vi "host.vi"() -> ()   [LabVIEW 2020]
uses:
  <vilib>/DAQmx/write.llb/DAQmx Write (Analog Wfm 1Chan NSamp).vi
  <vilib>/DAQmx/create/channels.llb/DAQmx Create Channel (AO-Voltage-Basic).vi
  <vilib>/DAQmx/configure/timing.llb/DAQmx Timing (Sample Clock).vi
  <vilib>/DAQmx/miscellaneous.llb/DAQmx Fill In Error Info.vi
  <vilib>/Utility/file.llb/Write Delimited Spreadsheet (DBL).vi
  <resource>/objmgr/daqmx.rc
panel:
  out "time":dbl
  in  "y predict save":path
  out "max iteration":dbl
  out "X":dbl[][](array[numeric])
  in  "X data filepath":path
  out "y waveform":cluster{"Numeric":dbl, "Double":dbl}(graph)
  in  "stop":bool
  out "iteration":dbl
  out "y predict values":dbl[](array[numeric])
  out "y":dbl[][](array[numeric])
  in  "y data filepath":path
  out "Waveform Graph":dbl[][](graph)
  out "t":dbl[][](array[numeric])
  in  "t data filepath":path
  out "size":dbl
  in  "error in":errorcluster
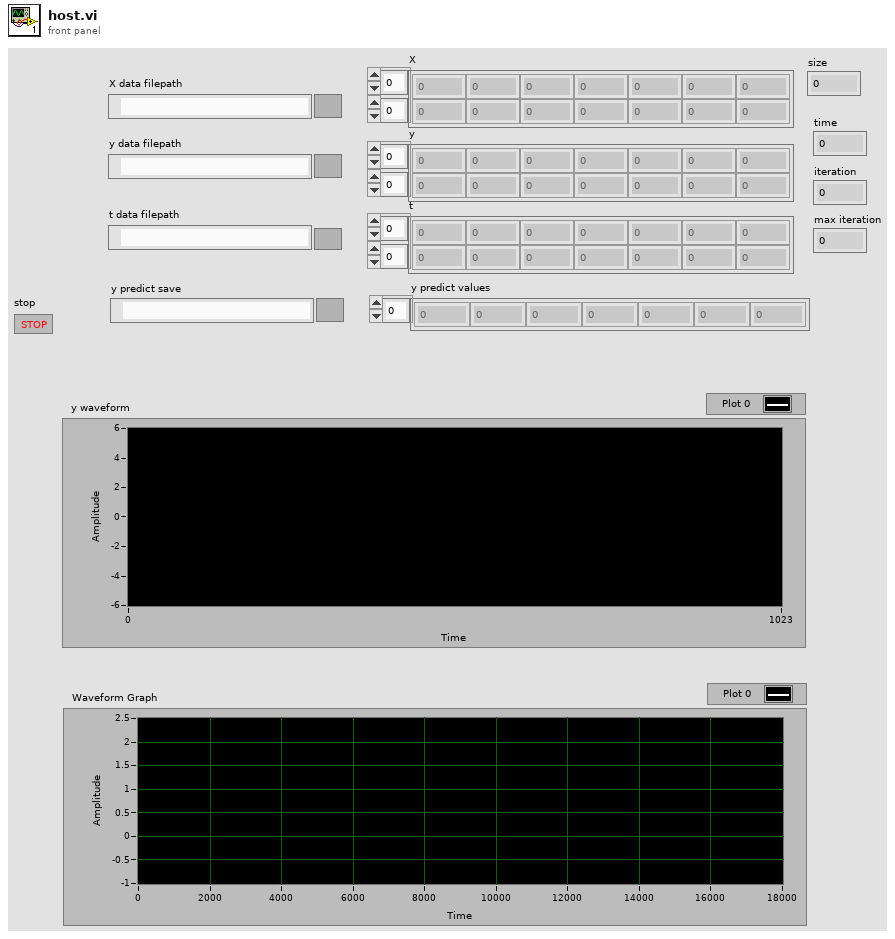
[diagram p1: front panel]
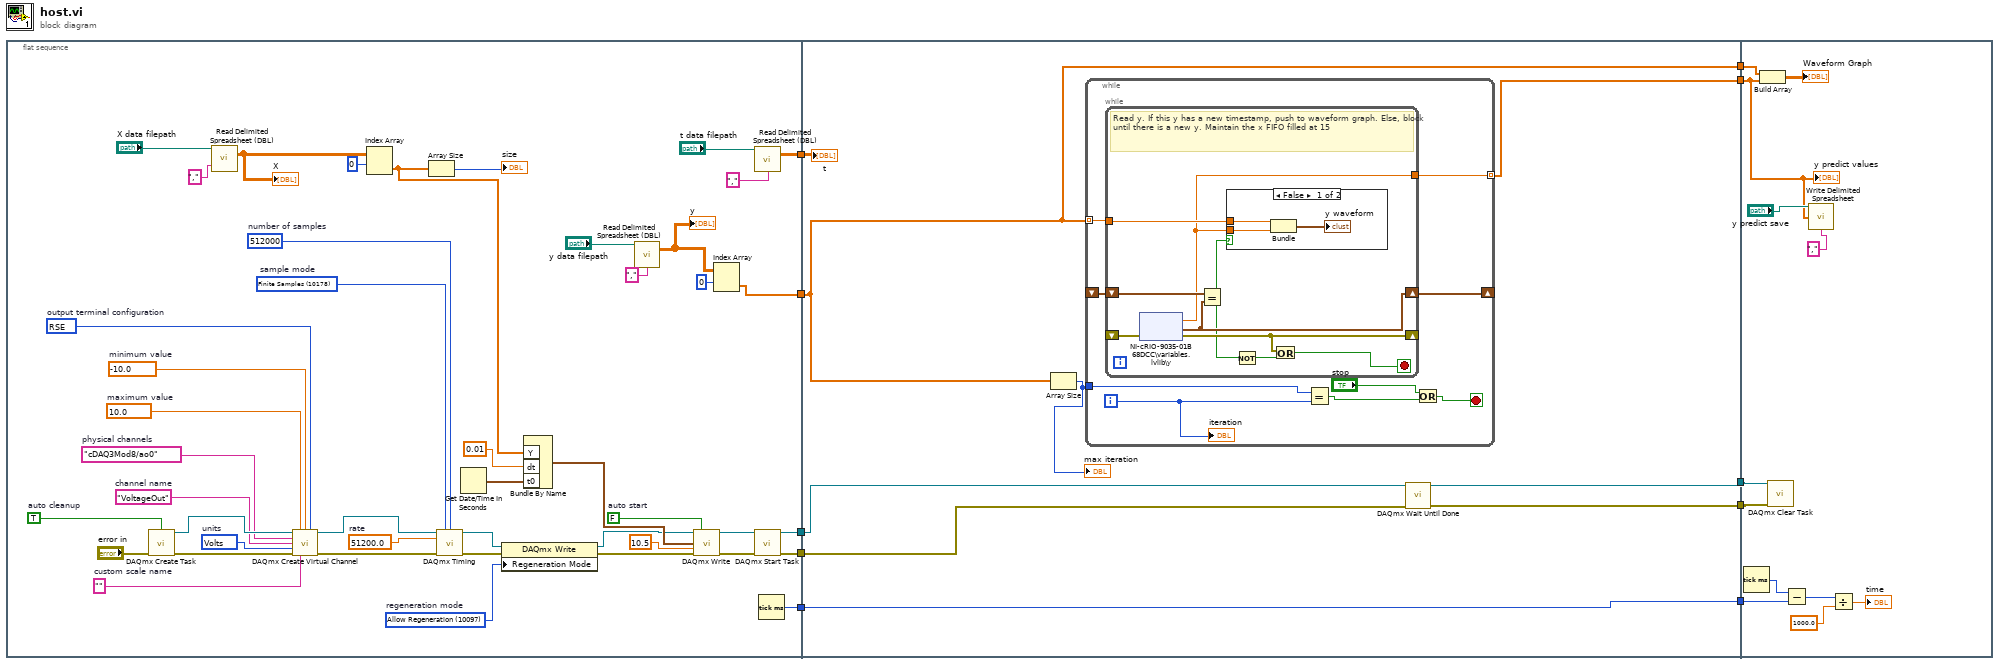
[diagram p0: block diagram]
diagram:
  n1 = flat-sequence {
    tunnel: [w53] -> w10
    tunnel: [w14] -> w9
    tunnel: [w13] -> w8
    tunnel: [w12] -> w6
    tunnel: [w11] -> w5
    tunnel: w10 -> [w64]
    tunnel: w9 -> [w56]
    tunnel: w8 -> [w57]
    tunnel: [w59] -> w7
    tunnel: w6 -> [w60]
    tunnel: w5 -> [w62]
    tunnel: [w62] -> w4
    tunnel: [w61] -> w3
    tunnel: [w60] -> w2
    tunnel: [w58] -> w1
    tunnel: w7 -> [w97]
    tunnel: w4 -> [w94]
    tunnel: w3 -> [w87]
    tunnel: w2 -> [w90]
    tunnel: w1 -> [w96]
    frame #0 {
      w21 = tag "cDAQ3Mod8/ao0"  # physical channels
      w26 = 512000  # number of samples
      w28 = 10097 items=["Allow Regeneration"=10097, "Do Not Allow Regeneration"=10158]  # regeneration mode
      w27 = 10178 items=["Finite Samples"=10178, "Continuous Samples"=10123, "Hardware Timed Single Point"=12522]  # sample mode
      w25 = 51200.0  # rate
      w22 = 10083 items=["Default"=-1, "RSE"=10083, "Differential"=10106, "Pseudodifferential"=12529]  # output terminal configuration
      w19 = 10348 items=["Volts"=10348, "From Custom Scale"=10065]  # units
      w20 = "VoltageOut"  # channel name
      w18 = ""  # custom scale name
      w23 = -10.0  # minimum value
      w24 = 10.0  # maximum value
      w17 = TRUE  # auto cleanup
      w16 = FALSE  # auto start
      n2 = call <vilib>:"DAQmx Create Task.vi"("auto cleanup"=w17, "error in"="error in") -> ("task out"=w34:refnum<k21>, "error out"=w33:errorcluster)  [unwired: 12 in]
      n3 = call <vilib>:"Read Delimited Spreadsheet (DBL).vi"("file path (dialog if empty)"="X data filepath", "delimiter (\\t)"=",") -> ("all rows"=w47:dbl[][])  [unwired: 8 in, 5 out]
      "X" <- w47
      n4 = call-poly <vilib>:"DAQmx Create Virtual Channel.vi"("task in"=w34, "maximum value"=w24, "minimum value"=w23, "output terminal configuration"=w22, "physical channels"=w21, "name to assign"=w20, "units"=w19, "error in"=w33, "custom scale name"=w18) -> ("task out"=w37:refnum<k21>, "error out"=w35:errorcluster)  [unwired: 5 in]
      n5 = Index Array(array=w47, index (row)=0) -> (element=w48:dbl[])  [unwired: 1 in]
      n6 = Array Size(array=w48) -> (size(s)=→"size":i32)
      n7 = call-poly <vilib>:"DAQmx Timing.vi"("task/channels in"=w37, "sample mode"=w27, "samples per channel"=w26, "rate"=w25, "error in"=w35) -> ("task out"=w38:refnum<k21>, "error out"=w36:errorcluster)  [unwired: 9 in]
      n8 = Get Date/Time In Seconds() -> (seconds since 1Jan1904=w43:timestamp)
      n9 = property class="DAQmx Write"(reference=w38, error in=w36, "Regeneration Mode"=w28) -> (reference out=w39:refnum<k21>, error out=w40:errorcluster)
      n10 = Bundle By Name("Y"=w48, "dt"=0.01, "t0"=w43) -> (w44:waveform(dbl))  [unwired: 1 in]
      n11 = call <vilib>:"Read Delimited Spreadsheet (DBL).vi"("file path (dialog if empty)"="y data filepath", "delimiter (\\t)"=",") -> ("all rows"=w51:dbl[][])  [unwired: 8 in, 5 out]
      "y" <- w51
      n12 = call-poly <vilib>:"DAQmx Write.vi"("task/channels in"=w39, "auto start"=w16, "data"=w44, "timeout"=10.5, "error in"=w40) -> ("task out"=w41:refnum<k21>, "error out"=w42:errorcluster)  [unwired: 8 in, 1 out]
      n13 = Index Array(array=w51, index (row)=0) -> (element=w12:dbl[])  [unwired: 1 in]
      n14 = call <vilib>:"Read Delimited Spreadsheet (DBL).vi"("file path (dialog if empty)"="t data filepath", "delimiter (\\t)"=",") -> ("all rows"=w53:dbl[][])  [unwired: 8 in, 5 out]
      n15 = call <vilib>:"DAQmx Start Task.vi"("task/channels in"=w41, "error in"=w42) -> ("task out"=w14:refnum<k21>, "error out"=w13:errorcluster)  [unwired: 12 in]
      n16 = Tick Count (ms)() -> (millisecond timer value=w11:u32)
    }
    frame #1 {
      n17 = Array Size(array=w60) -> (size(s)=w63:i32)
      "max iteration" <- w63
      n18 = while {
        tunnel: w60 -> [w73] mode=indexing
        tunnel: [w70] -> w61 mode=indexing
        shift-right: [w72] -> _
        shift-left: _ -> [w71]
        tunnel: w63 -> [w69]
        i -> [w65]
        stop <- w67 stop-if-true
        n19 = while {
          shift-right: [w81] -> w72
          shift-left: w71 -> [w80]
          shift-right: [w79] -> _
          shift-left: _ -> [w82]
          tunnel: w73 -> [w76]
          tunnel: [w75] -> w70
          stop <- w74 stop-if-true
          # "Read y. If this y has a new timestamp, push to waveform graph. Else, block until there is a new y. Maintain the x FIFO filled at 15"
          n20 = shared-variable "NI-cRIO-9035-01B68DCC\\variables.lvlib\\y"(error in=w82) -> (w75:dbl, error out=w79:errorcluster, w81:timestamp)
          n21 = Equal?(x=w80, y=w81) -> (x = y?=w77:bool)
          n22 = case shown="False" w77 {
            tunnel: w76 -> [w84 _]
            tunnel: w75 -> [w83 _]
            frame False {
              n23 = Bundle("Numeric"=w84, "Double"=w83) -> (→"y waveform":cluster{"Numeric":dbl, "Double":dbl})  [unwired: 1 in]
            }
            frame True {
            }
          }
          n24 = Not(x=w77) -> (.not. x?=w78:bool)
          n25 = Or(x=w79, y=w78) -> (x .or. y?=w74:bool)
        }
        n26 = Equal?(x=w69, y=w65) -> (x = y?=w66:bool)
        n27 = Or(x="stop", y=w66) -> (x .or. y?=w67:bool)
        "iteration" <- w65
      }
      n28 = call <vilib>:"DAQmx Wait Until Done.vi"("task/channels in"=w56, "error in"=w57) -> ("task out"=w59:refnum<k21>, "error out"=w58:errorcluster)  [unwired: 12 in]
      "t" <- w64
    }
    frame #2 {
      n29 = Tick Count (ms)() -> (millisecond timer value=w95:u32)
      n30 = Build Array(w90, w87) -> (→"Waveform Graph":dbl[][])
      n31 = call <vilib>:"DAQmx Clear Task.vi"("task in"=w97, "error in"=w96) -> ()  [unwired: 13 in, 1 out]
      n32 = Subtract(x=w95, y=w94) -> (x-y=w93:u32)
      n33 = call-poly <vilib>:"Write Delimited Spreadsheet.vi"("file path (dialog if empty)"="y predict save", "1D data"=w87, "delimiter (\\t)"=",") -> ()  [unwired: 11 in, 2 out]
      n34 = Divide(x=w93, y=1000.0) -> (x/y=→"time":dbl)
      "y predict values" <- w87
    }
  }
